vi "UserInfoManagerInit.vi"(8 "error in (no error)":errorcluster, 11 "userInfoManage in":refnum<class "UserInfoManageUI.lvclass">) -> (0 "error out":errorcluster, 3 "userInfoManage out":refnum<class "UserInfoManageUI.lvclass">)   [LabVIEW 2015, in "ActorManagement.lvlib" / "UserInfoManageUI.lvclass"]
uses:
  UserInfoManageUI.lvclass
  UserManagement/UserBasicInfo/UserBasicInfo.lvclass
  PluginWithDatabase/PluginWithDatabase.lvclass/PluginWithDatabase.ctl
  PluginWithDatabase/PluginWithDatabase.lvclass
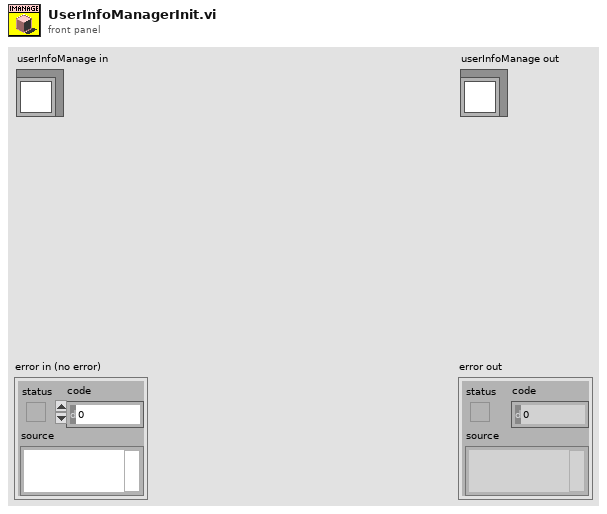
[diagram p1: front panel]
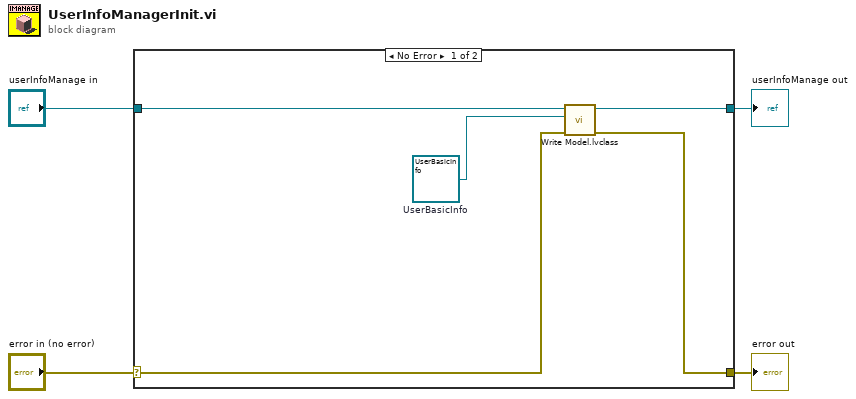
[diagram p0: block diagram]
diagram:
  n1 = case shown="No Error" "error in (no error)" {
    selector: "error in (no error)" -> [w7 w11]
    tunnel: [w6 w11] -> w3
    tunnel: [w8 w10] -> w1
    tunnel: "userInfoManage in" -> [w9 w10]
    frame No Error {
      w5 = refnum<class "UserBasicInfo.lvclass"> refnum  # UserBasicInfo
      n2 = call "Write Model.lvclass.vi"("error in (no error)"=w7, "UserManagement.lvlib:Model"=w5, "PluginWithDatabase in"=w9) -> ("error out"=w6:errorcluster, "PluginWithDatabase out"=w8:refnum<class "UserInfoManageUI.lvclass">)  [unwired: 7 in]
    }
    frame Error {
    }
  }
  "error out" <- w3
  "userInfoManage out" <- w1
